vi "Hardware-System-State-Host.vi"() -> ()   [LabVIEW 2016]
uses:
  <vilib>/Powertrain Controls/Device Drivers/DCM/Rev0/RT/System Settings.ctl
  <vilib>/Powertrain Controls/Device Drivers/DCM/Rev0/RT/User LED.ctl
  <vilib>/Powertrain Controls/Device Drivers/DCM/HH/RT/Duration Pre Scale.ctl
  <vilib>/Powertrain Controls/Device Drivers/DCM/Rev0/RT/System ADC.ctl
  <vilib>/Powertrain Controls/Device Drivers/DCM/Rev0/RT/Internal Fault.ctl
  Shared/Typedefs/System-ExpansionRIO-Setup.ctl
  Shared/Typedefs/System-ExpansionRIO-State.ctl
  <vilib>/Powertrain Controls/Device Drivers/DCM/Rev0/RT/DCM - RT.lvclass
  <vilib>/Powertrain Controls/Device Drivers/DCM/HH/RT/DCM - RT - HH.lvlib
  Shared/DSI-Shared.lvlib
panel:
  out "HW|DCM|ID":T1 {"Serial Number" format="%x"}
  in  "_System Settings":T2 {"HH Open Threshold [A]" min=0 max=8 format="%#_3p"; "HH ISeq Dur PS" items=["3.3ms @ 20MHz"=0, "6.5ms @ 10MHz"=4, "13ms @ 5MHz"=6, "26ms @ 2.5MHz"=7]; "HH Shoot Through Time [s]" min=0 max=0.003277 format="%#_3p"; "Clamp Fault Filter Time [s]" min=0 max=0.003277 format="%#_3p"; "DI HS Fault Filter Time [s]" min=0 max=0.003277 format="%#_3p"}
  in  "KeyThreshold":sgl caption="[V]"
  in  "UseKey":bool
  out "State":T7 caption="DCM System State" {"System ADC"."Fan [V]" format="%#_3p"; "System ADC"."Primary B1B2 [V]" format="%#_3p"; "System ADC"."Primary B3B4 [V]" format="%#_3p"; "System ADC"."Primary A3A4 [V]" format="%#_3p"; "System ADC"."Primary A1A2 [V]" format="%#_3p"; "System ADC"."MPRD [V]" format="%#_3p"; "System ADC"."Ext HV B [V]" format="%#_3p"; "System ADC"."Ext HV A [V]" format="%#_3p"; "System ADC"."Pump Zener B [V]" format="%#_3p"; "System ADC"."Pump Zener A [V]" format="%#_3p"; "System ADC"."DI Zener B [V]" format="%#_3p"; "System ADC"."DI Zener A [V]" format="%#_3p"; "System ADC"."Key [V]" format="%#_3p"; "System ADC"."DRVP [V]" format="%#_3p"; "System ADC"."Battery [V]" format="%#_3p"; "System ADC"."FET Driver [V]" format="%#_3p"; "System ADC"."Secondary B1B2 [V]" format="%#_3p"; "System ADC"."Secondary B3B4 [V]" format="%#_3p"; "System ADC"."Secondary A3A4 [V]" format="%#_3p"; "System ADC"."Secondary A1A2 [V]" format="%#_3p"; "System ADC"."Primary Range [V]" format="%#_3p"; "System ADC"."Temp Boost B [C]" format="%#_3p"; "System ADC"."Temp Primary A [C]" format="%#_3p"; "System ADC"."Temp Secondary A [C]" format="%#_3p"; "System ADC"."Temp Fan Intake [C]" format="%#_3p"; "System ADC"."Temp CPU [C]" format="%#_3p"; "System ADC"."Temp DI Zener B [C]" format="%#_3p"; "System ADC"."Temp DI B [C]" format="%#_3p"; "System ADC"."Temp DI Zener A [C]" format="%#_3p"; "System ADC"."Temp DI A [C]" format="%#_3p"; "System ADC"."Temp HH 7-12 [C]" format="%#_3p"; "System ADC"."Temp HH 1-6 [C]" format="%#_3p"; "System ADC"."AI 12 [V]" format="%#_3p"; "System ADC"."AI 11 [V]" format="%#_3p"; "System ADC"."AI 10 [V]" format="%#_3p"; "System ADC"."AI 9 [V]" format="%#_3p"; "System ADC"."AI 8 [V]" format="%#_3p"; "System ADC"."AI 7 [V]" format="%#_3p"; "System ADC"."AI 6 [V]" format="%#_3p"; "System ADC"."AI 5 [V]" format="%#_3p"; "System ADC"."AI 4 [V]" format="%#_3p"; "System ADC"."AI 3 [V]" format="%#_3p"; "System ADC"."AI 2 [V]" format="%#_3p"; "System ADC"."AI 1 [V]" format="%#_3p"}
  in  "_Hidden":enum32{"Invisible"}(tab)
  in  "MPRD":bool
  in  "HHOpenThreshold":sgl
  in  "HHISeqDurPS":u8
  in  "HHShootThroughTime":sgl
  in  "BleedFaultFilterTime":sgl
  in  "DI-HSFaultFilterTime":sgl
  in  "IOLockMPRDDisable":bool
  out "UserLED1":u8(ring) items=["Off", "Yellow", "Green"]
  out "UserLED2":u8(ring) items=["Off", "Yellow", "Green"]
  in  "HW|ExpansionRIO|Setup":T8
  out "HW|ExpansionRIO|State":T9
  # "DCM System Setup"
  # "DCM Identification"
  # "DCM System State"
  # "Personality Board / Expansion RIO Setup"
  # "Personality Board / Expansion RIO State"
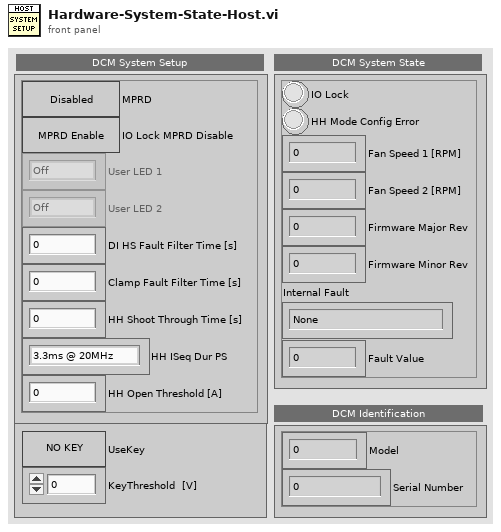
[diagram p1: front panel]
types:
  T1 = cluster{"Model":u16, "Rev Major":u8, "Rev Minor":u8, "Serial Number":u32}
  T2 = typedef "DCM - RT.lvclass/System Settings.ctl" = cluster{"MPRD":bool, "IO Lock MPRD Disable":bool, "User LED 1":T3, "User LED 2":T3, "DI HS Fault Filter Time [s]":sgl, "Clamp Fault Filter Time [s]":sgl, "HH Shoot Through Time [s]":sgl, "HH ISeq Dur PS":T4, "HH Open Threshold [A]":sgl}
  T3 = typedef "DCM - RT.lvclass/User LED.ctl" = enum16{"Off", "Yellow", "Green"}
  T4 = typedef "DCM - RT - HH.lvlib/Duration Pre Scale.ctl" = u8
  T5 = typedef "DCM - RT.lvclass/System ADC.ctl" = cluster{"AI 1 [V]":sgl, "AI 2 [V]":sgl, "AI 3 [V]":sgl, "AI 4 [V]":sgl, "AI 5 [V]":sgl, "AI 6 [V]":sgl, "AI 7 [V]":sgl, "AI 8 [V]":sgl, "AI 9 [V]":sgl, "AI 10 [V]":sgl, "AI 11 [V]":sgl, "AI 12 [V]":sgl, "Temp HH 1-6 [C]":sgl, "Temp HH 7-12 [C]":sgl, "Temp DI A [C]":sgl, "Temp DI Zener A [C]":sgl, "Temp DI B [C]":sgl, "Temp DI Zener B [C]":sgl, "Temp CPU [C]":sgl, "Temp Fan Intake [C]":sgl, "Temp Secondary A [C]":sgl, "Temp Primary A [C]":sgl, "Temp Boost B [C]":sgl, "Primary Range [V]":sgl, "Primary A1A2 [V]":sgl, "Primary A3A4 [V]":sgl, "Primary B3B4 [V]":sgl, "Primary B1B2 [V]":sgl, "Secondary A1A2 [V]":sgl, "Secondary A3A4 [V]":sgl, "Secondary B3B4 [V]":sgl, "Secondary B1B2 [V]":sgl, "Ext HV A [V]":sgl, "Ext HV B [V]":sgl, "FET Driver [V]":sgl, "Fan [V]":sgl, "Battery [V]":sgl, "DRVP [V]":sgl, "Key [V]":sgl, "DI Zener A [V]":sgl, "DI Zener B [V]":sgl, "Pump Zener A [V]":sgl, "Pump Zener B [V]":sgl, "MPRD [V]":sgl}
  T6 = typedef "DCM - RT.lvclass/Internal Fault.ctl" = enum32{"None", "Temp HH 1-6", "Temp HH 7-12", "Temp DI A", "Temp DI Zener A", "Temp DI B", "Temp DI Zener B", "Temp Intake", "Temp Primary A", "Temp Secondary A", "Temp Boost B", "Temp CPU", "Low Battery", "Inrush Protection", "A Run Enable", "B Run Enable"}
  T7 = cluster{"System ADC":T5, "IO Lock":bool, "HH Mode Config Error":bool, "Fan Speed 1 [RPM]":sgl, "Fan Speed 2 [RPM]":sgl, "Firmware Major Rev":u16, "Firmware Minor Rev":u16, "Internal Fault":T6, "Fault Value":dbl}
  T8 = typedef "DSI-Shared.lvlib/System-ExpansionRIO-Setup.ctl" = cluster{"Enable Expansion RIO":bool, "Bitfile":enum16{"Standard (NI 9149)", "Custom"}, "RIO Address":string, "Custom Bitfile Path":string}
  T9 = typedef "DSI-Shared.lvlib/System-ExpansionRIO-State.ctl" = cluster{"Error":bool, "Description":string}
  T10 = enum8{"Enabled", "Disabled", "Disabled and Grayed Out"}
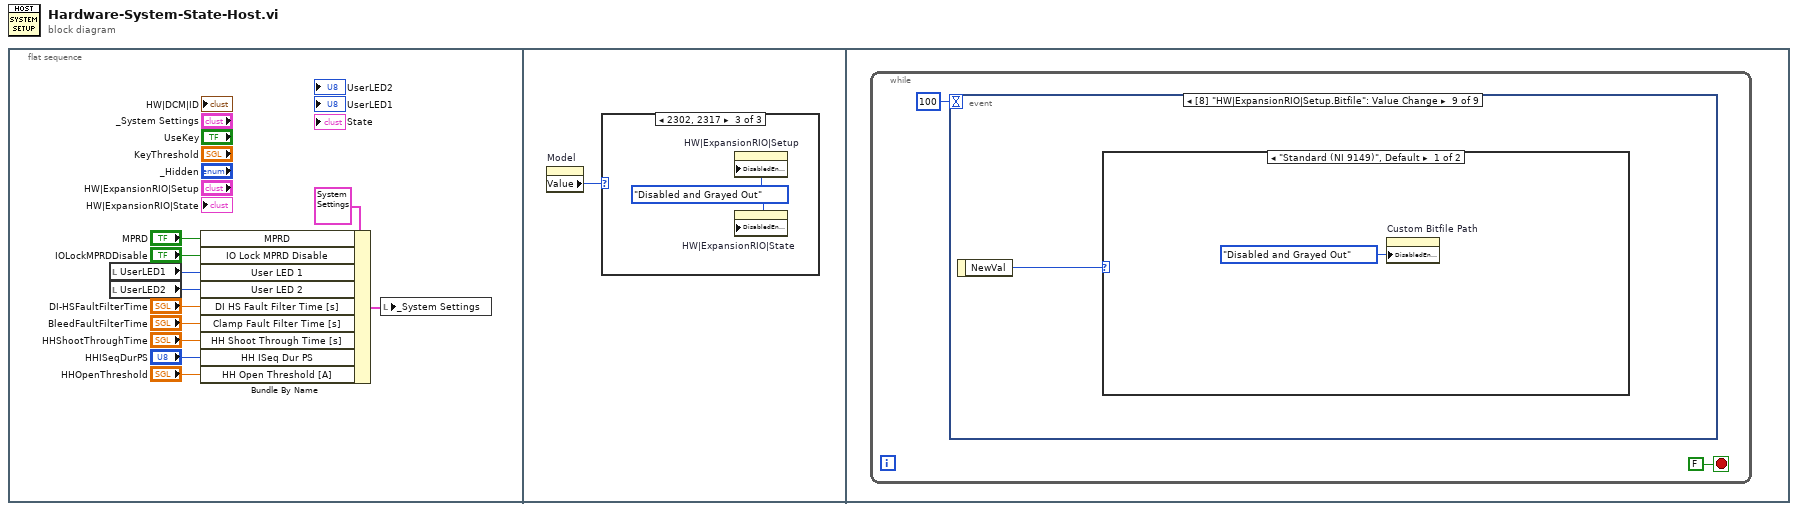
[diagram p0: block diagram]
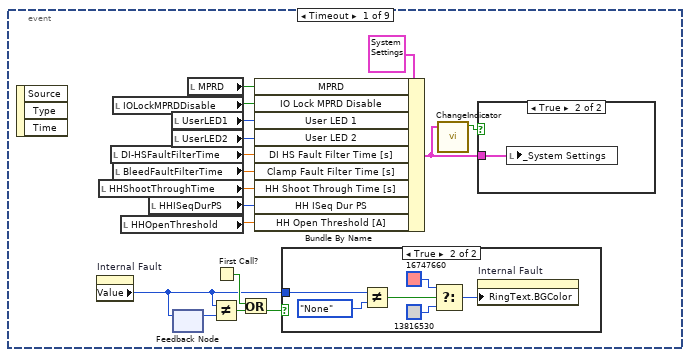
[diagram p4: hidden frame]
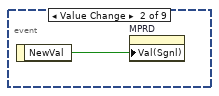
[diagram p7: hidden frame]
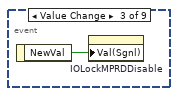
[diagram p8: hidden frame]
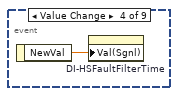
[diagram p9: hidden frame]
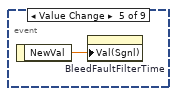
[diagram p10: hidden frame]
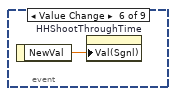
[diagram p11: hidden frame]
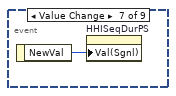
[diagram p12: hidden frame]
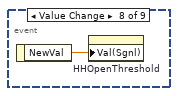
[diagram p13: hidden frame]
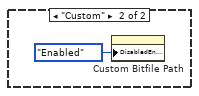
[diagram p14: hidden frame]
diagram:
  n1 = flat-sequence {
    frame #0 {
      n2 = local read "UserLED1"() -> (w2:u8)
      n3 = local read "UserLED2"() -> (w1:u8)
      n4 = Bundle By Name(cluster=T2 {"MPRD"=FALSE, "IO Lock MPRD Disable"=FALSE, "User LED 1"=enum."Off", "User LED 2"=enum."Off", "DI HS Fault Filter Time [s]"=0.0, "Clamp Fault Filter Time [s]"=0.0, "HH Shoot Through Time [s]"=0.0, "HH ISeq Dur PS"=0, "HH Open Threshold [A]"=0.0} ("_System Settings"), "MPRD"="MPRD", "IO Lock MPRD Disable"="IOLockMPRDDisable", "User LED 1"=w2, "User LED 2"=w1, "DI HS Fault Filter Time [s]"="DI-HSFaultFilterTime", "Clamp Fault Filter Time [s]"="BleedFaultFilterTime", "HH Shoot Through Time [s]"="HHShootThroughTime", "HH ISeq Dur PS"="HHISeqDurPS", "HH Open Threshold [A]"="HHOpenThreshold") -> (w3:T2)
      n5 = local write "_System Settings"(w3) -> ()
    }
    frame #1 {
      n6 = property on="Model" class="DigNum (strict)"() -> ("Value"=w12:u16)  [unwired: 2 in, 2 out]
      n7 = case shown="2302, 2317" w12 {
        frame Default {
        }
        frame 2301, 2316 {
        }
        frame 2302, 2317 {
          w13 = T10."Disabled and Grayed Out" ("Disabled")
          n8 = property on="HW|ExpansionRIO|Setup" class="Clust"("DisabledEnum"=w13) -> ()  [unwired: 2 in, 2 out]
          n9 = property on="HW|ExpansionRIO|State" class="Clust (strict)"("DisabledEnum"=w13) -> ()  [unwired: 2 in, 2 out]
        }
      }
    }
    frame #2 {
      n10 = while {
        stop <- FALSE stop-if-true
        n11 = event shown="[8] \"HW|ExpansionRIO|Setup.Bitfile\": Value Change" {
          selector: _ -> [_ _ _ _ _ _ _ _ _]
          dyn-events: _ -> [_ _ _ _ _ _ _ _ _]
          timeout: 100 -> [_ _ _ _ _ _ _ _ _]
          event Timeout {
            n12 = event-data() -> ()  [unwired: 1 in, 3 out]
            n13 = property on="Internal Fault" class="Enum (strict)"() -> ("Value"=w18:T6)  [unwired: 2 in, 2 out]
            n14 = local read "HHShootThroughTime"() -> (w27:sgl)
            n15 = local read "DI-HSFaultFilterTime"() -> (w29:sgl)
            n16 = local read "IOLockMPRDDisable"() -> (w30:bool)
            n17 = local read "BleedFaultFilterTime"() -> (w28:sgl)
            n18 = local read "HHOpenThreshold"() -> (w25:sgl)
            n19 = local read "HHISeqDurPS"() -> (w26:u8)
            n20 = local read "UserLED1"() -> (w16:u8)
            n21 = local read "UserLED2"() -> (w17:u8)
            n22 = feedback-in #1(w18) -> ()
            n23 = feedback #1() -> (w22:T6)  [unwired: 1 in]
            n24 = local read "MPRD"() -> (w31:bool)
            n25 = Not Equal?(x=w18, y=w22) -> (x != y?=w21:bool)
            n26 = First Call?() -> (First Call?: T/F=w19:bool)
            n27 = Or(x=w19, y=w21) -> (x .or. y?=w20:bool)
            n28 = Bundle By Name(cluster=T2 {"MPRD"=FALSE, "IO Lock MPRD Disable"=FALSE, "User LED 1"=enum."Off", "User LED 2"=enum."Off", "DI HS Fault Filter Time [s]"=0.0, "Clamp Fault Filter Time [s]"=0.0, "HH Shoot Through Time [s]"=0.0, "HH ISeq Dur PS"=0, "HH Open Threshold [A]"=0.0} ("_System Settings"), "MPRD"=w31, "IO Lock MPRD Disable"=w30, "User LED 1"=w16, "User LED 2"=w17, "DI HS Fault Filter Time [s]"=w29, "Clamp Fault Filter Time [s]"=w28, "HH Shoot Through Time [s]"=w27, "HH ISeq Dur PS"=w26, "HH Open Threshold [A]"=w25) -> (w23:T2)
            n29 = case shown="True" w20 {
              tunnel: w18 -> [_ w38]
              frame False {
              }
              frame True {
                n30 = Not Equal?(x=w38, y=Internal_Fault."None" ("Value")) -> (x != y?=w36:bool)
                n31 = Select(t=u32 16747660, s=w36, f=u32 13816530) -> (s? t:f=w33:u32)
                n32 = property on="Internal Fault" class="Enum (strict)"("RingText.BGColor"=w33) -> ()  [unwired: 2 in, 2 out]
              }
            }
            n33 = call "ChangeIndicator.vi"("Input"=w23) -> ("Change"=w24:bool)  [unwired: 9 in]
            n34 = case shown="True" w24 {
              tunnel: w23 -> [_ w39]
              frame False {
              }
              frame True {
                n35 = local write "_System Settings"(w39) -> ()
              }
            }
          }
          event Value Change {
            n36 = event-data() -> ("NewVal"=w40:bool)  [unwired: 1 in]
            n37 = property on="MPRD" class="Bool (strict)"("Val(Sgnl)"=w40) -> ()  [unwired: 2 in, 2 out]
          }
          event Value Change {
            n38 = event-data() -> ("NewVal"=w41:bool)  [unwired: 1 in]
            n39 = property on="IOLockMPRDDisable" class="Bool (strict)"("Val(Sgnl)"=w41) -> ()  [unwired: 2 in, 2 out]
          }
          event Value Change {
            n40 = event-data() -> ("NewVal"=w42:sgl)  [unwired: 1 in]
            n41 = property on="DI-HSFaultFilterTime" class="DigNum (strict)"("Val(Sgnl)"=w42) -> ()  [unwired: 2 in, 2 out]
          }
          event Value Change {
            n42 = event-data() -> ("NewVal"=w43:sgl)  [unwired: 1 in]
            n43 = property on="BleedFaultFilterTime" class="DigNum (strict)"("Val(Sgnl)"=w43) -> ()  [unwired: 2 in, 2 out]
          }
          event Value Change {
            n44 = event-data() -> ("NewVal"=w44:sgl)  [unwired: 1 in]
            n45 = property on="HHShootThroughTime" class="DigNum (strict)"("Val(Sgnl)"=w44) -> ()  [unwired: 2 in, 2 out]
          }
          event Value Change {
            n46 = event-data() -> ("NewVal"=w45:T4)  [unwired: 1 in]
            n47 = property on="HHISeqDurPS" class="DigNum (strict)"("Val(Sgnl)"=w45) -> ()  [unwired: 2 in, 2 out]
          }
          event Value Change {
            n48 = event-data() -> ("NewVal"=w46:sgl)  [unwired: 1 in]
            n49 = property on="HHOpenThreshold" class="DigNum (strict)"("Val(Sgnl)"=w46) -> ()  [unwired: 2 in, 2 out]
          }
          event Value Change {
            n50 = event-data() -> ("NewVal"=w47:enum16{"Standard (NI 9149)", "Custom"})  [unwired: 1 in]
            n51 = case shown="\"Standard (NI 9149)\", Default" w47 {
              frame "Standard (NI 9149)", Default {
                n52 = property on="Custom Bitfile Path" class="Str"("DisabledEnum"=T10."Disabled and Grayed Out" ("Disabled")) -> ()  [unwired: 2 in, 2 out]
              }
              frame "Custom" {
                n53 = property on="Custom Bitfile Path" class="Str"("DisabledEnum"=T10."Enabled" ("Disabled")) -> ()  [unwired: 2 in, 2 out]
              }
            }
          }
        }
      }
    }
  }
